vi "Load Voltage Sourcing and Measuring T12.vi"(0 "Vin SMU":refnum<k15>="Dev1") -> ()   [LabVIEW 2021, in "SMU T12.lvlib"]
doc: "Demonstrates how to use the DC Voltage Output Function to force an output voltage. This example initializes a session, configures the Output Function, Sense, Autorange, Voltage Level and Current Limit, initiates generation, waits for a specified delay, and measures the voltage and current output. This example uses Single Point source mode."
uses:
  SMU/SMU T12.lvlib
  Reusables/Resuables T12.lvlib
  SMU/controls/Configuration.ctl
  controls/Measurement Result T12.ctl
panel:
  in  "error in":errorcluster
  out "error out":errorcluster
  out "Voltage Measurement":T1 caption="Voltage Measurement (Attenuted)"
  out "Current Measurement":T1
  in  "Current Limit Range":dbl=0.01 format="%.3p"
  in  "Voltage Level Range":dbl=6.0 format="%.5p"
  in  "Current Limit":dbl=0.01 format="%.3p"
  in  "Voltage Level":dbl=2.0 format="%.5p"
  in  "Vin SMU Channel":string="0"
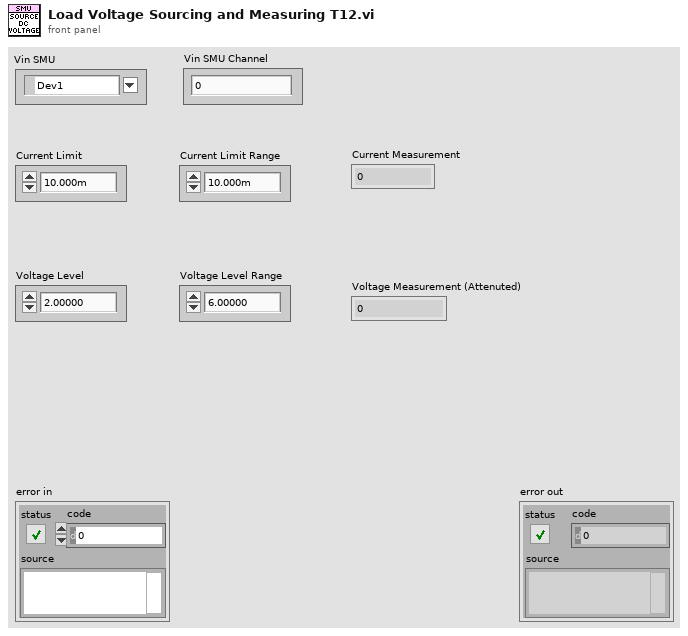
[diagram p1: front panel]
types:
  T1 = typedef "Measurement Result T12.ctl" = dbl
  T2 = typedef "Resuables T12.lvlib/Configuration.ctl" = cluster{"Voltage Level":dbl, "Voltage Level Range":dbl, "Current Limit":dbl, "Current Limit Range":dbl}
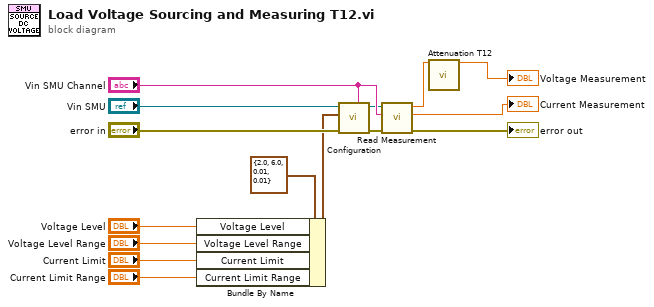
[diagram p0: block diagram]
diagram:
  n1 = Bundle By Name(cluster=T2 {"Voltage Level"=2.0, "Voltage Level Range"=6.0, "Current Limit"=0.01, "Current Limit Range"=0.01} ("Cluster"), "Voltage Level"="Voltage Level", "Voltage Level Range"="Voltage Level Range", "Current Limit"="Current Limit", "Current Limit Range"="Current Limit Range") -> (w3:T2)
  n2 = call "Configuration.vi"("Vin SMU Channel"="Vin SMU Channel", "error in (no error)"="error in", "Config"=w3, "IVI Refnum in"="Vin SMU") -> ("error out"=w5:errorcluster, "IVI Refnum out"=w6:refnum<k15>)  [unwired: 6 in]
  n3 = call "Read Measurement.vi"("error in (no error)"=w5, "Vin SMU Channel"="Vin SMU Channel", "IVI Refnum in"=w6) -> ("error out"=→"error out":errorcluster, "Current"=→"Current Measurement":dbl, "Voltage"=w2:dbl)  [unwired: 6 in]
  n4 = call "Attenuation T12.vi"("Measurement"=w2) -> ("Measurement Out"=→"Voltage Measurement":T1)  [unwired: 14 in]
